vi "PQunescapeBytea.vi"(8 "error in (no error)":errorcluster, 10 "retbuflen":u64, 11 "strtext":string) -> (0 "error out":errorcluster, 2 "PQunescapeBytea":string, 3 "retbuflen out":u64)   [LabVIEW 2019, in "libpqlv64.lvlib"]
uses:
  libpqlv64.lvlib
  libpq.dll
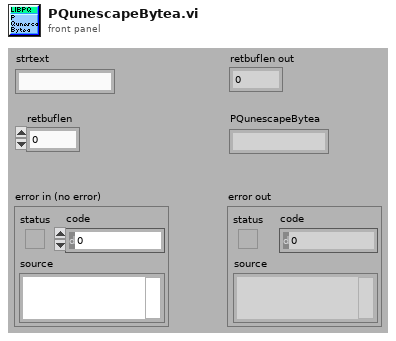
[diagram p1: front panel]
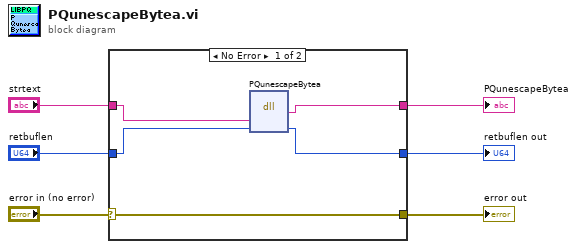
[diagram p0: block diagram]
diagram:
  n1 = case shown="No Error" "error in (no error)" {
    selector: "error in (no error)" -> [w11 w13]
    tunnel: [w11 w13] -> w5
    tunnel: [w10 _] -> w4
    tunnel: "strtext" -> [w9 _]
    tunnel: "retbuflen" -> [w8 w12]
    tunnel: [w7 w12] -> w1
    frame No Error {
      n2 = dll-call lib="libpq.*" fn="PQunescapeBytea"("strtext"=w9, "retbuflen"=w8) -> ("return type"=w10:string, "retbuflen"=w7:u64)  [unwired: 4 in, 2 out]
    }
    frame Error {
    }
  }
  "PQunescapeBytea" <- w4
  "retbuflen out" <- w1
  "error out" <- w5
